vi "TestExecuteTriggeredSubscription_PublishOK.vi"(8 "error in (no error)":errorcluster, 11 "TestCase in":refnum<class "TestSubscriptionPolicy.lvclass">) -> (0 "error out":errorcluster, 3 "TestCase out":refnum<class "TestSubscriptionPolicy.lvclass">)   [LabVIEW 2020, in "TestSubscriptionPolicy.lvclass"]
uses:
  TestSubscriptionPolicy.lvclass
  TestSubscriptionPolicy.lvclass/TestSubscriptionPolicy.ctl
  Source/IMediator/ISubscriptionPolicy/ISubscriptionPolicy.lvclass
  Source/SubscriptionPolicy/TriggeredSubscription/TriggeredSubscription.lvclass
  Source/SubscriptionPolicy/TriggeredSubscription/Trigger Condition.ctl
  modules/composed-transport/Source/Concrete/QueueTransport/QueueTransport.lvclass
  C:/Git/mva-core/modules/composed-transport/Source/ITransport/ITransport.lvclass
  C:/Git/mva-core/modules/composed-transport/Source/Concrete/QueueTransport/QueueTransport.lvclass
  C:/Git/mva-core/Source/IMediator/ISubscriptionPolicy/ISubscriptionPolicy.lvclass
  C:/Git/mva-core/Source/SubscriptionPolicy/TriggeredSubscription/TriggeredSubscription.lvclass
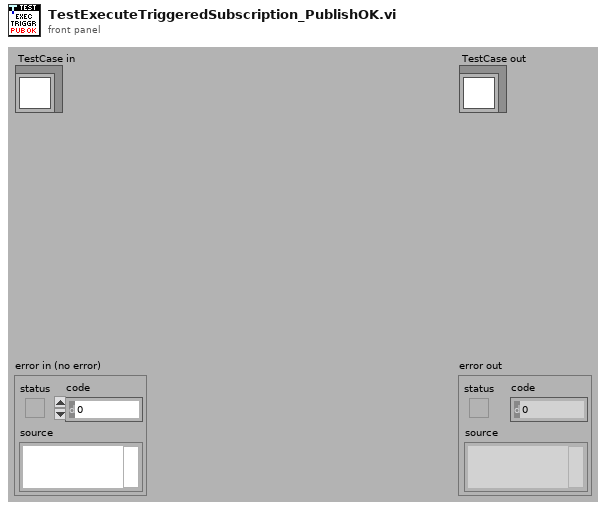
[diagram p1: front panel]
types:
  T1 = typedef "SubscriptionPolicy.lvlib/TriggeredSubscription.lvclass/Trigger Condition.ctl" = enum16{"Equal", "Not equal", "Greater than", "Less than", "Greater or equal", "Less or equal"}
  T2 = typedef "IMediator.lvlib/ISubscriptionPolicy.lvclass/ISubscriptionPolicy Reference.ctl" = refnum<data-value>
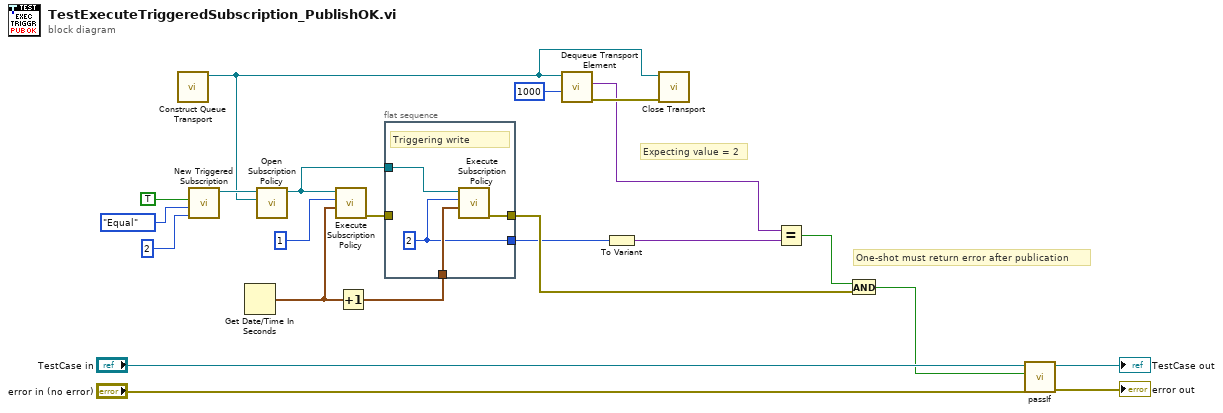
[diagram p0: block diagram]
diagram:
  # "One-shot must return error after publication"
  # "Expecting value = 2"
  n1 = call "Construct Queue Transport.vi"() -> ("QueueTransport"=w1:refnum<class "QueueTransport.lvclass">)  [unwired: 10 in, 1 out]
  n2 = call "New Triggered Subscription.vi"("Trigger Value"=2, "Trigger Condition"=Trigger_Condition."Equal", "Ignore Past Updates? (F)"=TRUE) -> ("TriggeredSubscription Out"=w16:refnum<class "TriggeredSubscription.lvclass">)  [unwired: 8 in]
  n3 = Get Date/Time In Seconds() -> (seconds since 1Jan1904=w7:timestamp)
  n4 = call "Open Subscription Policy.vi"("Transport"=w1, "SubscriptionPolicy"=w16) -> ("Subscription Policy"=w8:T2)  [unwired: 8 in, 1 out]
  n5 = call "Execute Subscription Policy.vi"("Publish Time"=w7, "New Topic Value"=1, "Subscription Policy"=w8) -> ("error out (Unsubscribe?)"=w3:errorcluster)  [unwired: 7 in, 1 out]
  n6 = Increment(x=w7) -> (x+1=w6:timestamp)
  n7 = flat-sequence {
    tunnel: w8 -> [w26]
    tunnel: w6 -> [w25]
    tunnel: [w24] -> w5
    tunnel: [w23] -> w4
    tunnel: w3 -> [_]
    frame #0 {
      w23 = 2
      # "Triggering write"
      n8 = call "Execute Subscription Policy.vi"("Publish Time"=w25, "New Topic Value"=w23, "Subscription Policy"=w26) -> ("error out (Unsubscribe?)"=w24:errorcluster)  [unwired: 7 in, 1 out]
    }
  }
  n9 = call "Dequeue Transport Element.vi"("Timeout In ms (-1)"=1000, "QueueTransport"=w1) -> ("error out"=w17:errorcluster, "Data"=w2:variant)  [unwired: 6 in, 2 out]
  n10 = To Variant(anything=w4) -> (Variant=w13:variant)
  n11 = call-dynamic "Close Transport.vi"("error in (no error)"=w17, "QueueTransport"=w1) -> ()  [unwired: 9 in, 1 out]
  n12 = Equal?(x=w2, y=w13) -> (x = y?=w12:bool)
  n13 = And(x=w12, y=w5) -> (x .and. y?=w11:bool)
  n14 = call-dynamic "passIf.vi"("error in (no error)"="error in (no error)", "pass"=w11, "TestCase in"="TestCase in") -> ("error out"=→"error out":errorcluster, "TestCase out"=→"TestCase out":refnum<class "TestSubscriptionPolicy.lvclass">)  [unwired: 7 in]
